vi "bcd to 7 segment decoder.vi"() -> ()   [LabVIEW 2018]
panel:
  out "g":bool
  out "f":bool
  out "e":bool
  out "d":bool
  out "c":bool
  out "b":bool
  out "a":bool
  in  "A":bool
  in  "B":bool
  in  "C":bool
  in  "D":bool
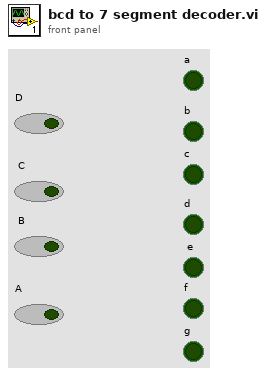
[diagram p1: front panel]
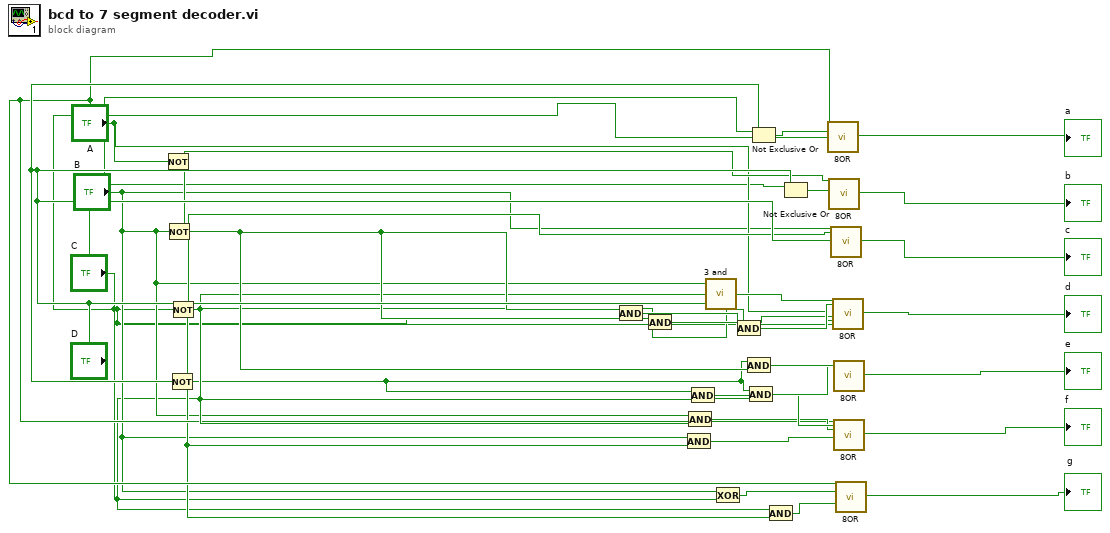
[diagram p0: block diagram]
diagram:
  n1 = Not(x="A") -> ()  [unwired: 1 out]
  n2 = Not(x="B") -> (.not. x?=w12:bool)
  n3 = Not(x="D") -> (.not. x?=w5:bool)
  n4 = Not(x="C") -> (.not. x?=w8:bool)
  n5 = And(x=w12, y="C") -> (x .and. y?=w14:bool)
  n6 = And(x=w12, y=w5) -> (x .and. y?=w15:bool)
  n7 = And(x="B", y=w5) -> (x .and. y?=w7:bool)
  n8 = And(x="B", y=w8) -> (x .and. y?=w9:bool)
  n9 = And(x=w5, y=w8) -> (x .and. y?=w10:bool)
  n10 = call "3 and.vi"("Boolean 3"="D", "Boolean 2"=w8, "Boolean"="B") -> ("Boolean 4"=w17:bool)
  n11 = Exclusive Or(1:"C", 2:"B") -> (0:w3:bool)
  n12 = And(x="C", y=w5) -> (x .and. y?=w16:bool)
  n13 = And(x=w5, y=w12) -> (x .and. y?=w13:bool)
  n14 = And(x=w5, y="C") -> (x .and. y?=w11:bool)
  n15 = Not Exclusive Or(1:"D", 2:"B") -> (0:w20:bool)
  n16 = And(x="C", y=w5) -> (x .and. y?=w4:bool)
  n17 = Not Exclusive Or(1:"D", 2:"C") -> (0:w19:bool)
  n18 = call "8OR.vi"("Boolean"="A", "Boolean 2"="C", "Boolean 3"=w20) -> ("Boolean 9"=→"a":bool)  [unwired: 24 in]
  n19 = call "8OR.vi"("Boolean"=w12, "Boolean 3"=w19) -> ("Boolean 9"=→"b":bool)  [unwired: 25 in]
  n20 = call "8OR.vi"("Boolean"="B", "Boolean 2"=w8, "Boolean 4"="D") -> ("Boolean 9"=→"c":bool)  [unwired: 24 in]
  n21 = call "8OR.vi"("Boolean"=w17, "Boolean 2"=w16, "Boolean 5"=w15, "Boolean 6"="A", "Boolean 7"=w14) -> ("Boolean 9"=→"d":bool)  [unwired: 22 in]
  n22 = call "8OR.vi"("Boolean"=w13, "Boolean 2"=w11) -> ("Boolean 9"=→"e":bool)  [unwired: 25 in]
  n23 = call "8OR.vi"("Boolean"="A", "Boolean 2"=w10, "Boolean 3"=w9, "Boolean 5"=w7) -> ("Boolean 9"=→"f":bool)  [unwired: 23 in]
  n24 = call "8OR.vi"("Boolean"="A", "Boolean 3"=w3, "Boolean 6"=w4) -> ("Boolean 9"=→"g":bool)  [unwired: 24 in]
